vi "GUI_laptop v15 loop time characterization.vi"() -> ()   [LabVIEW 2019]
uses:
  <vilib>/Math Plots/3D Math Plots/3D Scatter/3D Scatter XCtrl/3D Scatter.xctl
  <vilib>/Platform/TimedLoop/XDataNode/timing_clust.ctl
  <vilib>/Platform/TimedLoop/XDataNode/nitl_modes.ctl
  <vilib>/Platform/TimedLoop/XDataNode/wakeup.ctl
  <vilib>/Analysis/_algsub.llb/Real Vector Norm.vi
  <vilib>/Instr/_visa.llb/VISA Configure Serial Port (Instr).vi
  <vilib>/Utility/file.llb/Write Delimited Spreadsheet (DBL).vi
  <vilib>/addons/System Identification/Data Preprocess.llb/SI Lowpass Filter (MISO Array).vi
  <vilib>/Math Plots/3D Math Plots/3D Scatter/3D Scatter Datatype/Public/Plot Helper (Vector).vi
  <vilib>/platform/TimedLoop/XDataNode/XDataNode.xnode
  <vilib>/Platform/TimedLoop/XDataNode/XDNodeRunTimeDep.lvlib
  <vilib>/Analysis/NI_AALPro.lvlib
  <vilib>/Math Plots/3D Math Plots/3D Scatter/3D Scatter Datatype/3D Scatter Datatype.lvclass
  <vilib>/addons/System Identification/NI_SysID.lvlib
panel:
  out "Frame Duration 2":i64
  out "Frame Duration":i64
  out "Period":i64
  out "Finished Late? [i-1] 3":bool
  out "Actual End [i-1] 2":i64
  out "Expected End [i-1] 2":i64
  out "Actual End [i-1]":i64
  out "Expected End [i-1]":i64
  out "Finished Late? [i-1] 2":bool
  in  "Motion scale L3 outside rcm":dbl=2.0
  in  "L5 Deadzone":dbl
  in  "Sample rate":u32=500
  in  "Cutoff Frequency":dbl=10.0
  in  "Motion scale L1 L2":dbl=10.0
  in  "Motion scale L3":dbl=2.0
  in  "Save Path 4":path=path "C:/Users/jimmy/Documents/GitHub/Arduino-LabVIEW/zhantao/read_data_abs_filtered.csv"
  in  "Save Path 3":path=path "C:/Users/jimmy/Documents/GitHub/Arduino-LabVIEW/zhantao/read_data_abs_sending.csv"
  out "stimulus signals out":dbl[][](array[numeric]) format="%.2f"
  in  "L5 Offset":dbl
  in  "L5 Scale":dbl=1.0
  in  "Motion Scale L4":dbl=30.0
  out "spreadsheet string":string
  in  "Save Path 2":path=path "C:/Users/jimmy/Documents/GitHub/Arduino-LabVIEW/zhantao/read_data_delt.csv"
  out "send values":dbl[](array[numeric])
  out "Robot Feedback (l1 l2 l3 l4)":dbl[](array[numeric])
  in  "UDP Send":bool
  in  "UDP Recv":bool
  in  "L5 bound":dbl=1000.0
  in  "L4 bound (deg)":dbl=1000.0
  in  "L3 bound (mm)":dbl=1000.0
  in  "L2 bound (deg)":dbl=1000.0
  in  "L1 bound (deg)":dbl=1000.0
  in  "Joystick Type":dbl(ring)=1.0 items=["Rigid Joystick", "Free Joystick"]
  out "Finished Late? [i-1]":bool
  in  "Epsilon":dbl=0.2
  out "3D Scatter":refnum<class "3D Plot Datatype.lvclass">[](xcontrol)
  out "Random Point":dbl[](array[numeric])
  out "Virtual Cursor":dbl[](array[numeric])
  out "Iteration Duration":i64
  in  "Num of Points":i32=10
  in  "z bound":dbl=2.0
  in  "y bound":dbl=5.0
  in  "x bound":dbl=5.0
  in  "Stop":bool
  in  "Round Decimals":dbl=2.0 format="%#_15g"
  in  "Save Data":bool
  in  "Save Path":path=path "C:/Users/jimmy/Documents/GitHub/Arduino-LabVIEW/zhantao/read_data_abs.csv"
  in  "x speed":dbl=0.5
  in  "z speed":dbl=0.5
  in  "y speed":dbl=0.5
  out "error out":errorcluster
  in  "baud rate":u32=250000
  in  "VISA resource name":refnum<visa-resource-name>
  # "Other stuff"
  # "Reading Commands"
  # "Joystick Selection"
  # "Plotting"
  # "Data Saving"
  # "Arduino Communication"
  # "Master Slave Communication"
  # "Parameters"
  # "TODO: add a lowpass filter for l5"
  # "TODO: fix the bounds; currently bounds are arbitrary"
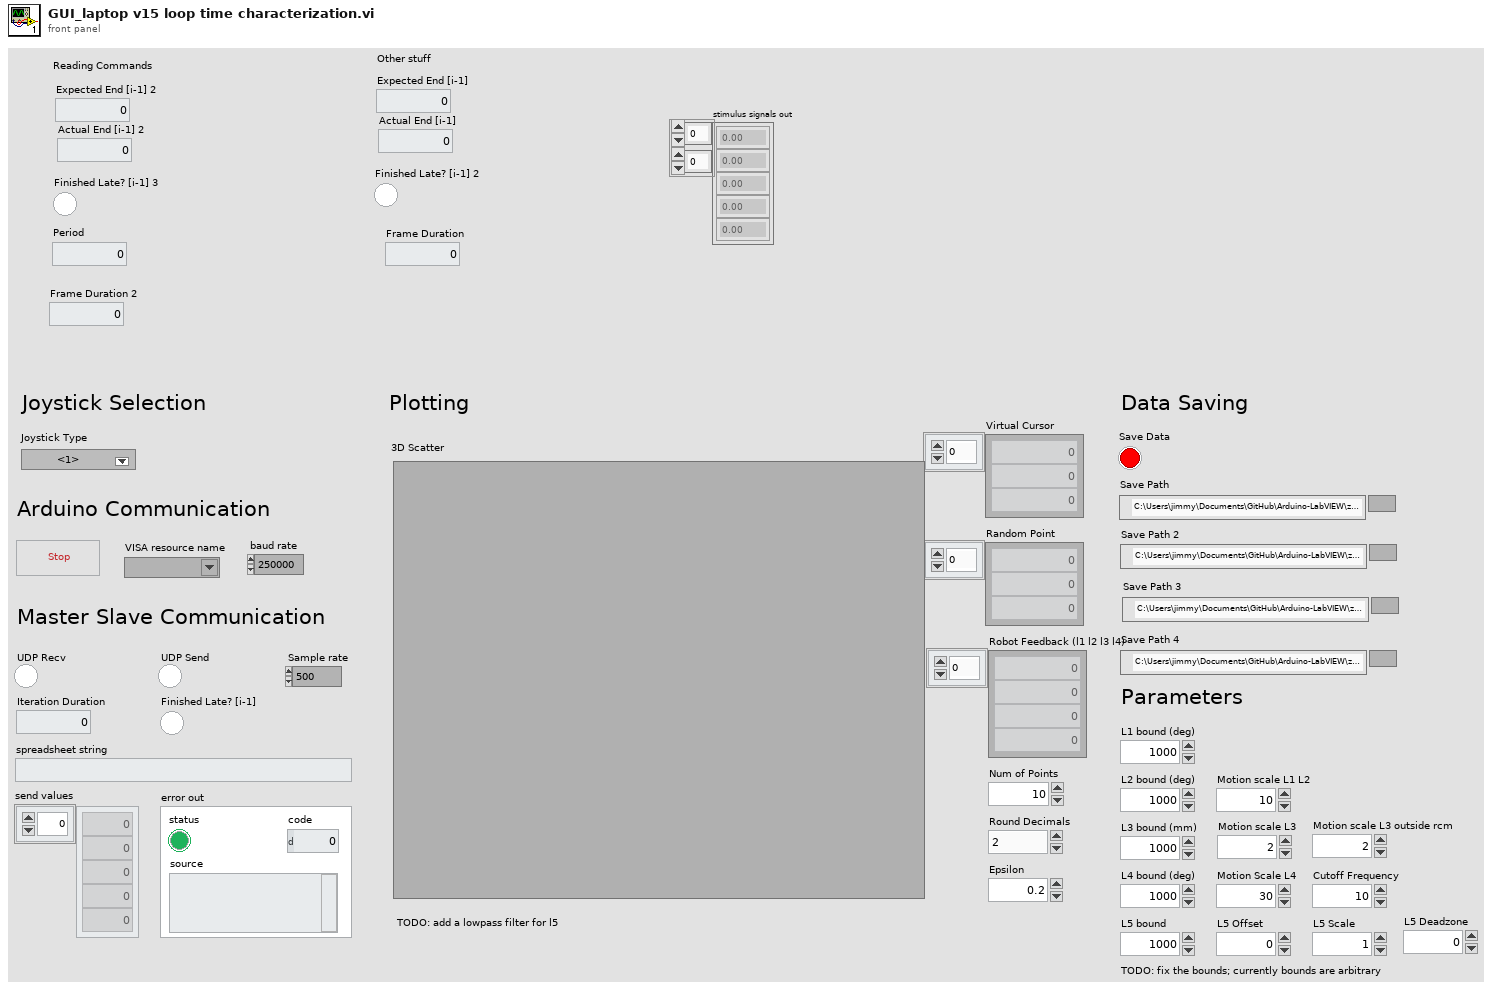
[diagram p1: front panel]
types:
  T1 = typedef "XDNodeRunTimeDep.lvlib/timing_clust.ctl" = cluster{"Expected End [f-1]":u64, "Actual End [f-1]":u64, "Finished Late? [f-1]":bool, "Expected End [i-1]":u64, "Actual End [i-1]":u64, "Finished Late? [i-1]":bool, "Expected Start [i]":u64, "Actual Start [i]":u64, "Expected Start [f]":u64, "Actual Start [f]":u64, "Source Name":string, "Structure Name":string, "Period":i64, "Deadline":i64, "Offset":i64, "Start":i64, "Priority":i32, "Timeout":i32, "Mode":T2, "Wakeup Reason":T3, "Error":errorcluster, "Source Type":string, "Secondary Source Type":string, "Global End Time":u64, "Global Start Time":u64, "Frame Duration":u64, "Iteration Duration":u64, "Assigned CPU":i32, "I/O Scan Engine Mode":u32}
  T2 = typedef "XDNodeRunTimeDep.lvlib/nitl_modes.ctl" = enum32{"No Change", "Process missed periods, maintain original phase", "Discard missed periods, maintain original phase", "Process missed periods, ignore original phase", "Discard missed periods, ignore original phase"}
  T3 = typedef "XDNodeRunTimeDep.lvlib/wakeup.ctl" = enum32{"Normal", "Aborted", "Asynchronous wakeup", "Timing source error", "Timed loop error", "Timeout"}
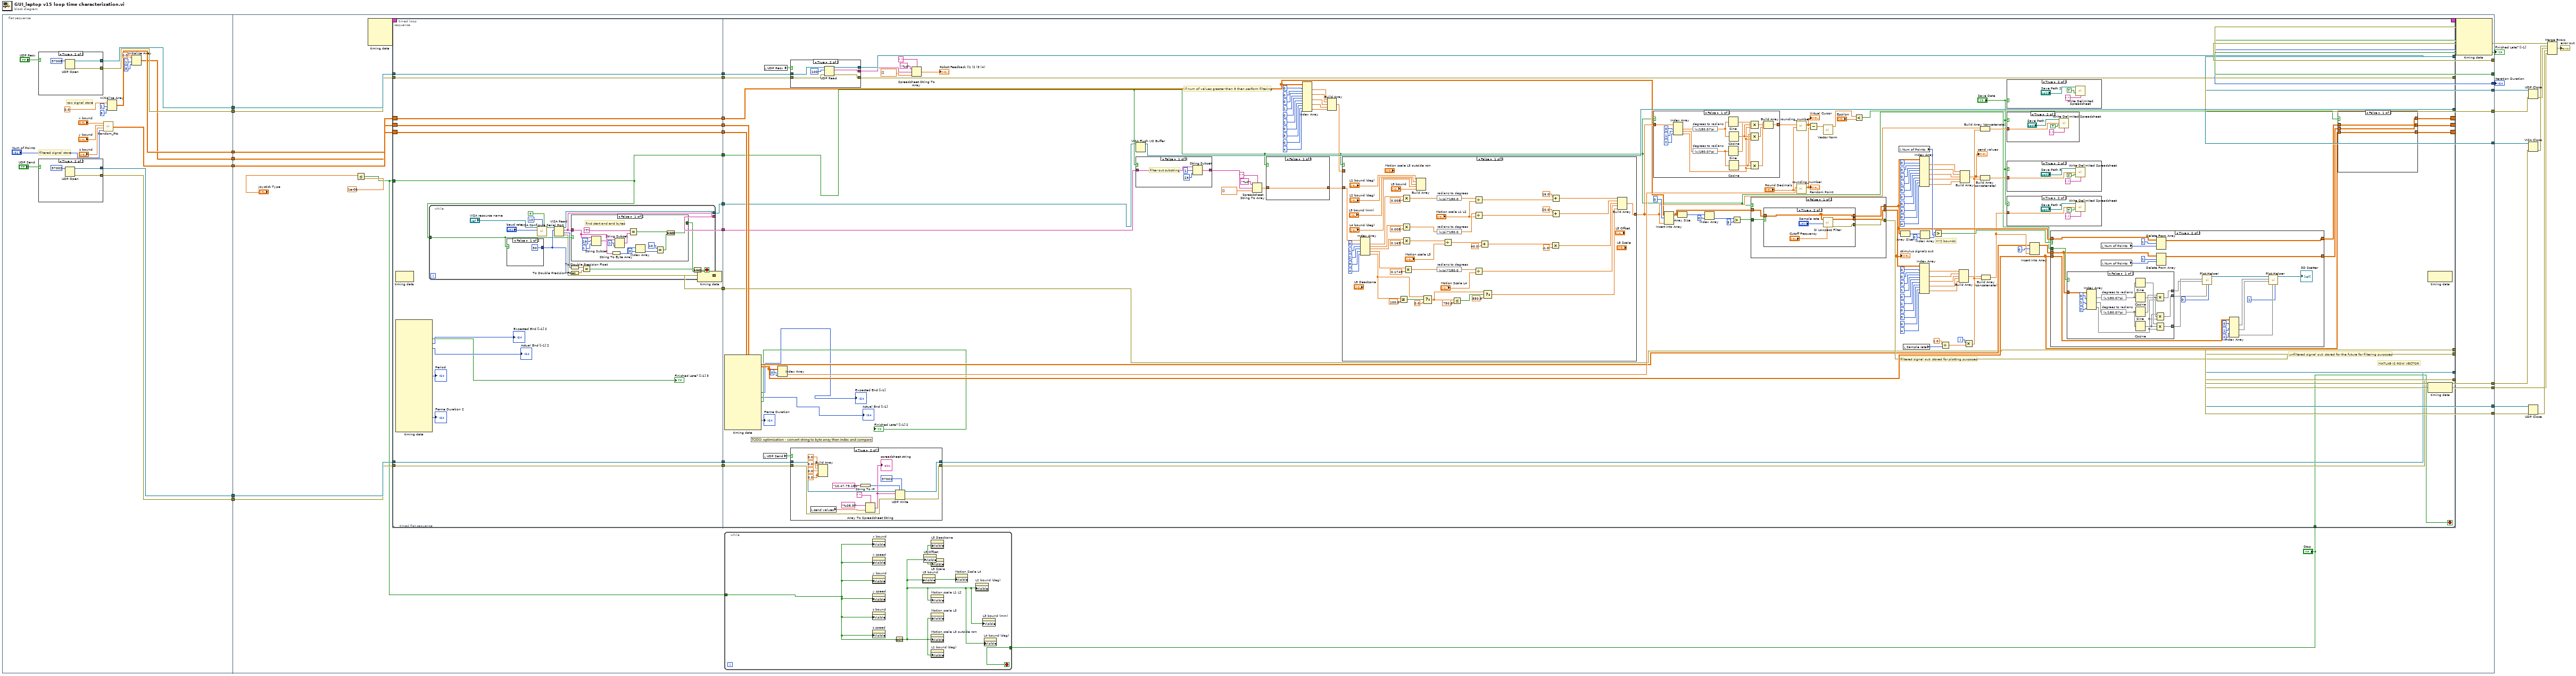
[diagram p0: block diagram]
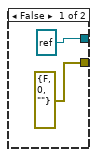
[diagram p2: hidden frame]
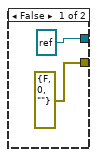
[diagram p3: hidden frame]
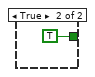
[diagram p4: hidden frame]
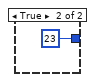
[diagram p5: hidden frame]
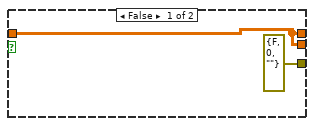
[diagram p8: hidden frame]
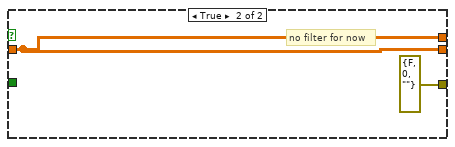
[diagram p9: hidden frame]
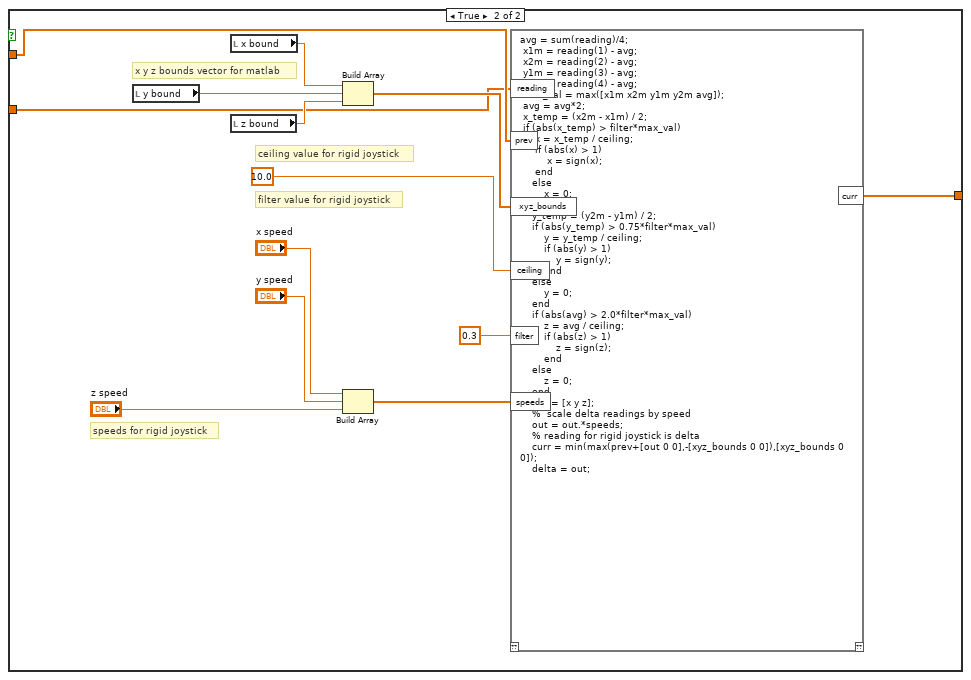
[diagram p10: hidden frame]
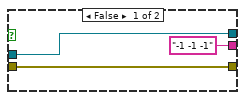
[diagram p13: hidden frame]
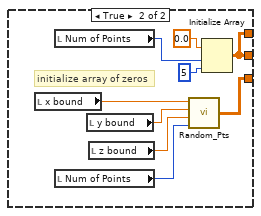
[diagram p15: hidden frame]
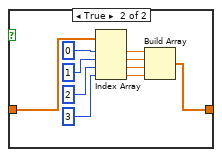
[diagram p17: hidden frame]
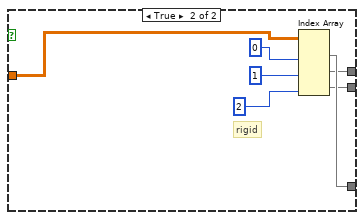
[diagram p20: hidden frame]
diagram:
  n1 = flat-sequence {
    tunnel: [w32] -> w18
    tunnel: [w36] -> w17
    tunnel: [w31] -> w16
    tunnel: [w30] -> w15
    tunnel: [w27] -> w14
    tunnel: [w26] -> w13
    tunnel: [w22] -> w2
    tunnel: [w71] -> w21
    tunnel: [w70] -> w20
    tunnel: [w68] -> w12
    tunnel: [w66] -> w19
    tunnel: w18 -> [w69]
    tunnel: w17 -> [w67]
    tunnel: w16 -> [w65]
    tunnel: w15 -> [w64]
    tunnel: w14 -> [w63]
    tunnel: w13 -> [w62]
    tunnel: [w61] -> w6
    tunnel: [w60] -> w11
    tunnel: [w59] -> w5
    tunnel: [w58] -> w4
    tunnel: [w57] -> w3
    tunnel: w2 -> [w56]
    tunnel: [w55] -> w1
    frame #0 {
      # "filtered signal store"
      # "raw signal store"
      n2 = case shown="True" "UDP Recv" {
        tunnel: [refnum<k16> refnum ("port") w49] -> w30
        tunnel: [errorcluster {"status"=FALSE, "code"=0, "source"=""} ("error out") w48] -> w27
        frame False {
        }
        frame True {
          n3 = UDP Open(11:u16 37008 ("port")) -> (port=w49:refnum<k16>, 0:w48:errorcluster)  [unwired: 4 in, 1 out]
        }
      }
      n4 = case shown="True" "UDP Send" {
        tunnel: [refnum<k16> refnum ("port") w44] -> w31
        tunnel: [errorcluster {"status"=FALSE, "code"=0, "source"=""} ("error out") w43] -> w26
        frame False {
        }
        frame True {
          n5 = UDP Open(11:u16 37002 ("port")) -> (port=w44:refnum<k16>, 0:w43:errorcluster)  [unwired: 4 in, 1 out]
        }
      }
      n6 = call "Random_Pts.vi"("Num of Points"="Num of Points", "z bound"="z bound", "y bound"="y bound", "x bound"="x bound") -> ("appended array"=w36:dbl[][])
      n7 = Initialize Array(0.0 ("element"), 1 ("dimension size"), 5 ("dimension size")) -> (w32:dbl[][])
      n8 = Initialize Array(0.0 ("element"), 1 ("dimension size"), 5 ("dimension size")) -> (w22:dbl[][])
    }
    frame #1 {
      n9 = Less Or Equal?(x="Joystick Type", y=1e-06) -> (x <= y?=w51:bool)
      n10 = node-c288() -> (w73:T1)  [unwired: 4 in]
      n11 = timed-loop {
        tunnel: [w95] -> w71
        tunnel: [w94] -> w70
        shift-right: [w83] -> _
        shift-left: w69 -> [w84]
        timing: w73 -> [_]
        timing-out: [_] -> w72
        shift-right: [w81] -> _
        shift-left: w67 -> [w82]
        tunnel: w65 -> [w93]
        tunnel: w64 -> [w92]
        tunnel: w63 -> [w91]
        tunnel: w62 -> [w90]
        tunnel: [w89] -> w61
        tunnel: [w88] -> w60
        tunnel: [w87] -> w59
        tunnel: [w86] -> w58
        tunnel: [w85] -> w57
        shift-right: [w79] -> _
        shift-left: w56 -> [w80]
        tunnel: "Stop" -> [w78]
        tunnel: w51 -> [w77]
        i -> [w199]
        stop <- w183 stop-if-true
        n12 = timed-sequence {
          timing: _ -> [_]
          timing-out: _ -> [_]
          tunnel: [w125] -> w95
          tunnel: [w124] -> w94
          tunnel: w93 -> [w123]
          tunnel: w92 -> [w122]
          tunnel: w91 -> [w121]
          tunnel: w90 -> [w120]
          tunnel: [w119] -> w89
          tunnel: [w118] -> w88
          tunnel: [w117] -> w87
          tunnel: [w116] -> w86
          tunnel: [w115] -> w85
          tunnel: w84 -> [w114]
          tunnel: [w113] -> w83
          tunnel: w82 -> [w112]
          tunnel: [w111] -> w81
          tunnel: w80 -> [w110]
          tunnel: [w109] -> w79
          tunnel: w78 -> [w97]
          tunnel: w77 -> [w96]
          n13 = timed-flat-sequence {
            tunnel: w110 -> [w135]
            tunnel: w112 -> [w136]
            tunnel: w114 -> [w137]
            tunnel: w120 -> [w138]
            tunnel: w121 -> [w139]
            tunnel: w122 -> [w140]
            tunnel: w123 -> [w141]
            tunnel: [w141] -> w108
            tunnel: [w140] -> w107
            tunnel: [w139] -> w106
            tunnel: [w138] -> w105
            tunnel: [w137] -> w104
            tunnel: [w136] -> w103
            tunnel: [w135] -> w102
            tunnel: [w134] -> w101
            tunnel: [w133] -> w100
            tunnel: [w132] -> w99
            tunnel: [w128] -> w98
            tunnel: w96 -> [w128]
            tunnel: [w254] -> w125
            tunnel: [w185] -> w124
            tunnel: [w262] -> w119
            tunnel: [w261] -> w118
            tunnel: [w260] -> w117
            tunnel: [w259] -> w116
            tunnel: [w244] -> w115
            tunnel: [w305] -> w113
            tunnel: [w301] -> w111
            tunnel: [w201] -> w109
            tunnel: w108 -> [w267]
            tunnel: w107 -> [w266]
            tunnel: w106 -> [w264]
            tunnel: w105 -> [w263]
            tunnel: w104 -> [w209]
            tunnel: w103 -> [w302]
            tunnel: w102 -> [w204]
            tunnel: w101 -> [w190]
            tunnel: w100 -> [w189]
            tunnel: w99 -> [w185]
            tunnel: w98 -> [w184]
            tunnel: w97 -> [w183]
            frame #0 {
              n14 = node-c288() -> (→"Finished Late? [i-1] 3":bool, →"Expected End [i-1] 2":i64, →"Actual End [i-1] 2":i64, →"Period":i64, →"Frame Duration 2":i64)  [unwired: 1 in, 18 out]
              n15 = while {
                tunnel: [w142] -> w133
                tunnel: [w155] -> w132
                tunnel: [w149] -> w134
                tunnel: w128 -> [w143]
                stop <- w145 stop-if-true
                n16 = case shown="False" w143 {
                  tunnel: [30 u32 23 ("byte count")] -> w148
                  frame False {
                  }
                  frame True {
                  }
                }
                n17 = call-poly "VISA Configure Serial Port"("VISA resource name"="VISA resource name", "termination char\n(0xA = '\\n' = LF)"=u8 10 ("termination char\n(0xA = '\\n' = LF)"), "Enable Termination\nChar (T)"=TRUE ("Enable Termination\nChar (T)"), "baud rate (9600)"="baud rate") -> ("VISA resource name out"=w150:refnum<visa-resource-name>)  [unwired: 10 in, 1 out]
                n18 = VISA Read(VISA resource name=w150, byte count=w148) -> (VISA resource name out=w149:refnum<visa-resource-name>, read buffer=w142:string, return count=w157:u32, error out=w155:errorcluster)  [unwired: 1 in]
                n19 = To Double Precision Float(number=w157) -> (double precision float=w156:dbl)
                n20 = To Double Precision Float(number=w148) -> (double precision float=w147:dbl)
                n21 = case shown="False" w143 {
                  tunnel: [w164 TRUE] -> w144
                  tunnel: w142 -> [w167 _]
                  frame False {
                    # "find start and end bytes"
                    n22 = String Subset(string=w167, offset (0)=29, length (rest)=1) -> (substring=w162:string)
                    n23 = String To Byte Array(string=w162) -> (unsigned byte array=w161:u8[])
                    n24 = String Subset(string=w167, length (rest)=1) -> (substring=w170:string)  [unwired: 1 in]
                    n25 = Equal?(x="T", y=w170) -> (x = y?=w166:bool)
                    n26 = Index Array(array=w161, index=0) -> (element=w159:u8)
                    n27 = Equal?(x=10, y=w159) -> (x = y?=w165:bool)
                    n28 = And(x=w166, y=w165) -> (x .and. y?=w164:bool)
                  }
                  frame True {
                  }
                }
                n29 = Equal?(x=w156, y=w147) -> (x = y?=w146:bool)
                n30 = And(x=w146, y=w144) -> (x .and. y?=w145:bool)
              }
              n31 = node-c288() -> ()  [unwired: 1 in, 1 out]
            }
            frame #1 {
              # "unfiltered signal out; stored for the future for filtering purposes"
              # "filtered signal out; stored for plotting purposes"
              # "XYZ bounds"
              # "if num of values greater than 5 then perform filtering"
              # "MATLAB IS ROW VECTOR"
              n32 = node-c288() -> (→"Expected End [i-1]":i64, →"Actual End [i-1]":i64, →"Finished Late? [i-1] 2":bool, →"Frame Duration":i64)  [unwired: 1 in, 11 out]
              n33 = local read "UDP Send"() -> (w194:bool)
              n34 = local read "UDP Recv"() -> (w265:bool)
              n35 = Index Array(array=w302, index (col)=0 ("index (row)")) -> (element=w276:dbl[])  [unwired: 1 in]
              n36 = case shown="True" w265 {
                tunnel: w266 -> [w413 w420]
                tunnel: w264 -> [w414 w419]
                tunnel: [w414 w418] -> w262
                tunnel: [w413 w417] -> w260
                tunnel: ["-1 -1 -1" w415] -> w255
                frame False {
                }
                frame True {
                  n37 = UDP Read(connection ID=w420, max size (548)=100, 8:w419) -> (data out=w415:string, error out=w418:errorcluster, 3:w417:refnum<k16>)  [unwired: 1 in, 2 out]
                }
              }
              n38 = case shown="True" w194 {
                tunnel: w267 -> [w395 w411]
                tunnel: w263 -> [w396 w407]
                tunnel: [w396 w403] -> w261
                tunnel: [w395 w402] -> w259
                frame False {
                }
                frame True {
                  w401 = 0.0 ("element")
                  n39 = local read "send values"() -> (w397:dbl[])
                  n40 = Build Array(0.0 ("element"), 0.0 ("element"), 0.0 ("element"), w401, w401) -> ()  [unwired: 1 out]
                  n41 = String To IP(1:"10.47.79.181" ("name")) -> (0:w405:u32)
                  n42 = Array To Spreadsheet String(delimiter (Tab)=" ", array=w397, 3:"%08.3f" ("format string")) -> (spreadsheet string=w408:string)
                  "spreadsheet string" <- w408
                  n43 = UDP Write(address=w405, port or service name=u16 37001, connection ID=w411, data in=w408, 8:w407) -> (error out=w403:errorcluster, 3:w402:refnum<k16>)  [unwired: 1 in]
                }
              }
              n44 = Spreadsheet String To Array(delimiter (Tab)=" ", format string="%d", spreadsheet string=w255, array type (2D Dbl)=dbl[] []) -> (array=→"Robot Feedback (l1 l2 l3 l4)":dbl[])
              n45 = VISA Flush I/O Buffer(VISA resource name=w190) -> (VISA resource name out=w254:refnum<visa-resource-name>)  [unwired: 2 in, 1 out]
              n46 = case shown="False" w184 {
                tunnel: w189 -> [w440 w441]
                tunnel: [w437 w441] -> w277
                frame False {
                  # "filter out substring"
                  n47 = String Subset(string=w440, offset (0)=1, length (rest)=29) -> (substring=w437:string)
                }
                frame True {
                }
              }
              n48 = Spreadsheet String To Array(delimiter (Tab)=",", format string="%d", spreadsheet string=w277, array type (2D Dbl)=dbl[] []) -> (array=w278:dbl[])
              n49 = case shown="False" w184 {
                tunnel: w278 -> [w442 w446]
                tunnel: [w442 w445] -> w252
                frame False {
                }
                frame True {
                  n50 = Index Array(array=w446, index #1=0 ("Plot ID"), index #2=1 ("Plot ID"), index #3=2 ("Plot ID"), index #4=3 ("index")) -> (element #1=w449:dbl, element #2=w448:dbl, element #3=w447:dbl, element #4=w443:dbl)
                  n51 = Build Array(w449, w448, w447, w443) -> (w445:dbl[])
                }
              }
              n52 = Index Array(array=w209, index (row) #1=0 ("disabled index (row)"), index (col) #1=0 ("disabled index (col)"), index (row) #2=0 ("disabled index (row)"), index (col) #2=1 ("disabled index (col)"), index (row) #3=0 ("disabled index (row)"), index (col) #3=2 ("disabled index (col)"), index (row) #4=0 ("disabled index (row)"), index (col) #4=3 ("disabled index (col)"), index (row) #5=0 ("disabled index (row)"), index (col) #5=4 ("disabled index (col)")) -> (element #1=w287:dbl, element #2=w286:dbl, element #3=w285:dbl, element #4=w280:dbl, element #5=w279:dbl)
              n53 = Build Array(w287, w286, w285, w280, w279) -> (w253:dbl[])
              n54 = case shown="False" w184 {
                tunnel: w253 -> [_ w381]
                tunnel: w252 -> [w368 w380]
                tunnel: [w328 w379] -> w228
                frame False {
                  n55 = Index Array(array=w368, index #1=0 ("Plot ID"), index #2=1 ("Plot ID"), index #3=2 ("Plot ID"), index #4=3 ("Plot ID"), index #5=4 ("Plot ID")) -> (element #1=w367:dbl, element #2=w355:dbl, element #3=w347:dbl, element #4=w345:dbl, element #5=w337:dbl)
                  n56 = Greater Or Equal?(x=w337, y=100.0) -> (x >= y?=w335:bool)
                  n57 = Multiply(x=w367, y=0.005) -> (x*y=w363:dbl)
                  n58 = Multiply(x=w355, y=0.005) -> (x*y=w358:dbl)
                  n59 = Multiply(x=w347, y=0.163) -> (x*y=w351:dbl)
                  n60 = Multiply(x=w345, y=0.1745) -> (x*y=w344:dbl)
                  n61 = Build Array("L1 bound (deg)", "L2 bound (deg)", "L3 bound (mm)", "L4 bound (deg)", "L5 bound") -> ()  [unwired: 1 out]
                  n62 = Select(t=w337, s=w335, f=0.0) -> (s? t:f=w330:dbl)
                  n63 = expression code="(x/pi)*180.0" "radians to degrees"(w363) -> (w362:dbl)
                  n64 = expression code="(x/pi)*180.0" "radians to degrees"(w358) -> (w357:dbl)
                  n65 = expression code="(x/pi)*180.0" "radians to degrees"(w344) -> (w343:dbl)
                  n66 = Divide(x=w351, y="Motion scale L3") -> (x/y=w349:dbl)
                  n67 = Less Or Equal?(x=w330, y=750.0) -> (x <= y?=w331:bool)
                  n68 = Divide(x=w362, y="Motion scale L1 L2") -> (x/y=w365:dbl)
                  n69 = Divide(x=w357, y="Motion scale L1 L2") -> (x/y=w360:dbl)
                  n70 = Divide(x=w343, y="Motion Scale L4") -> (x/y=w338:dbl)
                  n71 = Add(x=w349, y=40.0) -> (x+y=w353:dbl)
                  n72 = Select(t=w330, s=w331, f=850.0) -> (s? t:f=w329:dbl)
                  n73 = Multiply(x=w353, y=-1.0) -> (x*y=w339:dbl)
                  n74 = Add(x=16.0, y=w365) -> (x+y=w341:dbl)
                  n75 = Add(x=20.0, y=w360) -> (x+y=w340:dbl)
                  n76 = Build Array(w341, w340, w339, w338, w329) -> (w328:dbl[])
                }
                frame True {
                  # "ceiling value for rigid joystick"
                  # "filter value for rigid joystick"
                  # "speeds for rigid joystick"
                  # "x y z bounds vector for matlab"
                  n77 = local read "y bound"() -> (w390:dbl)
                  n78 = local read "x bound"() -> (w389:dbl)
                  n79 = local read "z bound"() -> (w391:dbl)
                  n80 = Build Array(w389, w390, w391) -> (w382:dbl[])
                  n81 = Build Array("x speed", "y speed", "z speed") -> (w385:dbl[])
                  n82 = script code="avg = sum(reading)/4;\n x1m = reading(1) - avg;\n x2m = reading(2) - avg;\n y1m = reading(3) - avg;\n y2m = reading(4) - avg;\n max_val = max([x1m x2m y1m y2m avg]);\n avg = avg*2;\n x_temp = (x2m - x1m) / 2;\n if (abs(x_temp) > filter*max_val)\n     x = x_temp / ceiling;\n     if (abs(x) > 1)\n         x = sign(x);\n     end\n    else\n        x = 0;\n    end\n    y_temp = (y2m - y1m) / 2;\n    if (abs(y_temp) > 0.75*filter*max_val)\n        y = y_temp / ceiling;\n        if (abs(y) > 1)\n            y = sign(y);\n        end\n    else\n        y = 0;\n    end\n    if (abs(avg) > 2.0*filter*max_val)\n        z = avg / ceiling;\n        if (abs(z) > 1)\n            z = sign(z);\n        end\n    else\n        z = 0;\n    end\n    out = [x y z];\n    %  scale delta readings by speed\n    out = out.*speeds;\n    % reading for rigid joystick is delta\n    curr = min(max(prev+[out 0 0],-[xyz_bounds 0 0]),[xyz_bounds 0 0]);\n    delta = out;"("xyz_bounds"=w382, "ceiling"=10.0 ("Real"), "filter"=0.3 ("Real"), "speeds"=w385, "reading"=w380, "prev"=w381) -> ("curr"=w379:dbl[])  [unwired: 1 in, 1 out]
                }
              }
              n83 = case shown="False" w184 {
                tunnel: [w466 w470] -> w303
                tunnel: w228 -> [w465 w470]
                frame False {
                  n84 = Index Array(array=w465, index #1=0 ("Plot ID"), index #2=1 ("Plot ID"), index #3=2 ("Plot ID")) -> (element #1=w464:dbl, element #2=w463:dbl, element #3=w453:dbl)
                  n85 = expression code="(x/180.0)*pi" "degrees to radians"(w464) -> (w462:dbl)
                  n86 = expression code="(x/180.0)*pi" "degrees to radians"(w463) -> (w461:dbl)
                  n87 = Sine(x=w462) -> (sin(x)=w459:dbl)
                  n88 = Sine(x=w461) -> (sin(x)=w458:dbl)
                  n89 = Cosine(x=w462) -> (cos(x)=w455:dbl)
                  n90 = Cosine(x=w461) -> (cos(x)=w456:dbl)
                  n91 = Compound Arithmetic op=MULTIPLY(w458, w455, w453) -> (w457:dbl)
                  n92 = Compound Arithmetic op=MULTIPLY(w456, w455, w453) -> (w454:dbl)
                  n93 = Compound Arithmetic op=MULTIPLY(w459, w456, w453) -> (w460:dbl)
                  n94 = Build Array(w460, w457, w454) -> (w466:dbl[])
                }
                frame True {
                }
              }
              n95 = Insert Into Array(array=w209, index (row)=0, new element=w228) -> (w245:dbl[][])  [unwired: 1 in]
              n96 = Array Size(array=w245) -> (size(s)=w248:i32[])
              n97 = Index Array(array=w248, index=0) -> (element=w247:i32)
              n98 = Greater?(x=w247, y=5) -> (0:w195:bool)
              n99 = case shown="False" w184 {
                tunnel: w195 -> [w316 _]
                tunnel: w245 -> [w318 w326]
                tunnel: [w317 w326] -> w207
                tunnel: [w315 errorcluster {"status"=FALSE, "code"=0, "source"=""} ("error out")] -> w244
                tunnel: [w314 w326] -> w210
                frame False {
                  n100 = case shown="True" w316 {
                    tunnel: w318 -> [w319 w324]
                    tunnel: [w319 w324] -> w317
                    tunnel: [errorcluster {"status"=FALSE, "code"=0, "source"=""} ("error out") w325] -> w315
                    tunnel: [w319 w323] -> w314
                    frame False {
                    }
                    frame True {
                      n101 = call-poly <vilib>:"SI Lowpass Filter.vi"("cutoff frequency"="Cutoff Frequency", "sampling rate (Hz)"="Sample rate", "stimulus signals in"=w324) -> ("error out"=w325:errorcluster, "stimulus signals out"=w323:dbl[][])  [unwired: 6 in, 1 out]
                    }
                  }
                }
                frame True {
                  # "no filter for now"
                }
              }
              "stimulus signals out" <- w210
              n102 = call "rounding_number.vi"("power of ten"="Round Decimals", "Array"=w303) -> ("rounded"=w274:dbl[])  [unwired: 9 in]
              "Virtual Cursor" <- w274
              n103 = call "rounding_number.vi"("power of ten"="Round Decimals", "Array"=w276) -> ("rounded"=w273:dbl[])  [unwired: 9 in]
              "Random Point" <- w273
              n104 = Subtract(x=w274, y=w273) -> (x-y=w272:dbl[])
              n105 = call-poly <vilib>:"Vector Norm.vi"("Input Vector"=w272) -> ("norm"=w271:dbl)  [unwired: 9 in, 1 out]
              n106 = Less?(x=w271, y="Epsilon") -> (x < y?=w269:bool)
              n107 = local read "Num of Points"() -> (w289:i32)
              n108 = Array Size(array=w207) -> (size(s)=w251:i32[])
              n109 = local read "Sample rate"() -> (w196:u32)
              n110 = Index Array(array=w207, index (row) #1=0 ("disabled index (col)"), index (col) #1=0 ("disabled index (row)"), index (row) #2=0 ("disabled index (col)"), index (col) #2=1 ("disabled index (row)"), index (row) #3=0 ("disabled index (col)"), index (col) #3=2 ("disabled index (row)"), index (row) #4=0 ("disabled index (col)"), index (col) #4=3 ("disabled index (row)"), index (row) #5=0 ("disabled index (col)"), index (col) #5=4 ("disabled index (col)")) -> (element #1=w233:dbl, element #2=w232:dbl, element #3=w231:dbl, element #4=w230:dbl, element #5=w229:dbl)
              n111 = Index Array(array=w210, index (row) #1=0 ("disabled index (col)"), index (col) #1=0 ("disabled index (row)"), index (row) #2=0 ("disabled index (col)"), index (col) #2=1 ("disabled index (row)"), index (row) #3=0 ("disabled index (col)"), index (col) #3=2 ("disabled index (row)"), index (row) #4=0 ("disabled index (col)"), index (col) #4=3 ("disabled index (row)"), index (row) #5=0 ("disabled index (col)"), index (col) #5=4 ("disabled index (col)")) -> (element #1=w216:dbl, element #2=w215:dbl, element #3=w214:dbl, element #4=w213:dbl, element #5=w212:dbl)
              n112 = Index Array(array=w251, index=0) -> (element=w290:i32)
              n113 = Greater?(x=w290, y=w289) -> (0:w288:bool)
              n114 = Divide(x=1.0, y=w196) -> (x/y=w197:dbl)
              n115 = Build Array(w216, w215, w214, w213, w212) -> (w193:dbl[])
              n116 = Build Array(w233, w232, w231, w230, w229) -> (w192:dbl[])
              "send values" <- w192
              n117 = Multiply(x=w199, y=w197) -> (x*y=w200:dbl)
              n118 = Build Array (concatenate)(w228, w200) -> (w227:dbl[])
              n119 = Build Array (concatenate)(w192, w200) -> (w208:dbl[])
              n120 = Build Array (concatenate)(w193, w200) -> (w205:dbl[])
              n121 = case shown="True" "Save Data" {
                frame False {
                }
                frame True {
                  n122 = call-poly <vilib>:"Write Delimited Spreadsheet.vi"("file path (dialog if empty)"="Save Path 2", "append to file? (new file:F)"=TRUE, "delimiter (\\t)"="," ("delimiter (\\t)")) -> ()  [unwired: 11 in, 2 out]
                }
              }
              n123 = case shown="True" "Save Data" {
                tunnel: w227 -> [_ w421]
                frame False {
                }
                frame True {
                  n124 = call-poly <vilib>:"Write Delimited Spreadsheet.vi"("file path (dialog if empty)"="Save Path", "1D data"=w421, "append to file? (new file:F)"=TRUE, "delimiter (\\t)"="," ("delimiter (\\t)")) -> ()  [unwired: 10 in, 2 out]
                }
              }
              n125 = case shown="True" "Save Data" {
                tunnel: w208 -> [_ w310]
                frame False {
                }
                frame True {
                  n126 = call-poly <vilib>:"Write Delimited Spreadsheet.vi"("file path (dialog if empty)"="Save Path 3", "1D data"=w310, "append to file? (new file:F)"=TRUE, "delimiter (\\t)"="," ("delimiter (\\t)")) -> ()  [unwired: 10 in, 2 out]
                }
              }
              n127 = case shown="True" "Save Data" {
                tunnel: w205 -> [_ w306]
                frame False {
                }
                frame True {
                  n128 = call-poly <vilib>:"Write Delimited Spreadsheet.vi"("file path (dialog if empty)"="Save Path 4", "1D data"=w306, "append to file? (new file:F)"=TRUE, "delimiter (\\t)"="," ("delimiter (\\t)")) -> ()  [unwired: 10 in, 2 out]
                }
              }
              n129 = Insert Into Array(array=w204, index (row)=0, new element=w205) -> (w203:dbl[][])  [unwired: 1 in]
              n130 = case shown="True" w288 {
                tunnel: w207 -> [w472 w494]
                tunnel: [w472 w493] -> w304
                tunnel: w302 -> [w471 w492]
                tunnel: w184 -> [_ w477]
                tunnel: w203 -> [_ w474]
                tunnel: [w471 w473] -> w202
                frame False {
                }
                frame True {
                  n131 = case shown="False" w477 {
                    tunnel: w474 -> [w511 w515]
                    tunnel: [w498 w514] -> w483
                    tunnel: [w497 w513] -> w482
                    tunnel: [w496 w512] -> w481
                    frame False {
                      n132 = Index Array(array=w511, index (col) #1=0 ("Plot ID"), index (col) #2=1 ("Plot ID"), index (col) #3=2 ("Plot ID")) -> (element #1=w501:dbl[], element #2=w500:dbl[], element #3=w499:dbl[])  [unwired: 3 in]
                      n133 = expression code="(x/180.0)*pi" "degrees to radians"(w501) -> (w507:dbl[])
                      n134 = expression code="(x/180.0)*pi" "degrees to radians"(w500) -> (w506:dbl[])
                      n135 = Sine(x=w507) -> (sin(x)=w505:dbl[])
                      n136 = Cosine(x=w507) -> (cos(x)=w502:dbl[])
                      n137 = Sine(x=w506) -> (sin(x)=w504:dbl[])
                      n138 = Cosine(x=w506) -> (cos(x)=w503:dbl[])
                      n139 = Compound Arithmetic op=MULTIPLY(w504, w502, w499) -> (w497:dbl[])
                      n140 = Compound Arithmetic op=MULTIPLY(w503, w502, w499) -> (w496:dbl[])
                      n141 = Compound Arithmetic op=MULTIPLY(w505, w503, w499) -> (w498:dbl[])
                    }
                    frame True {
                      # "rigid"
                      n142 = Index Array(array=w515, index (col) #1=0 ("disabled index (col)"), index (col) #2=1 ("index (col)"), index (col) #3=2 ("index (col)")) -> (element #1=w514:dbl[], element #2=w513:dbl[], element #3=w512:dbl[])  [unwired: 3 in]
                    }
                  }
                  n143 = local read "Num of Points"() -> (w491:i32)
                  n144 = local read "Num of Points"() -> (w476:i32)
                  n145 = Delete From Array(array=w494, length=1, index (row)=w491) -> (array with subset deleted=w493:dbl[][])  [unwired: 1 in, 1 out]
                  n146 = Delete From Array(array=w474, length=1, index (row)=w476) -> (array with subset deleted=w473:dbl[][])  [unwired: 1 in, 1 out]
                  n147 = call-poly <vilib>:"Plot Helper.vi"("Plot ID"=0, "z vector"=w481, "y vector"=w482, "x vector"=w483) -> ("3D Plot lvclass Array out"=w485:refnum<class "3D Plot Datatype.lvclass">[])  [unwired: 2 in, 5 out]
                  n148 = Index Array(array=w492, index (row) #1=0 ("index (row)"), index (row) #2=1 ("index (row)"), index (row) #3=2 ("index (row)")) -> (element #1=w489:dbl[], element #2=w488:dbl[], element #3=w487:dbl[])  [unwired: 3 in]
                  n149 = call-poly <vilib>:"Plot Helper.vi"("Plot ID"=1, "z vector"=w487, "y vector"=w488, "x vector"=w489, "3D Plot lvclass Array in"=w485) -> ("3D Plot lvclass Array out"=→"3D Scatter":refnum<class "3D Plot Datatype.lvclass">[])  [unwired: 1 in, 5 out]
                }
              }
              n150 = case shown="False" w269 {
                tunnel: w302 -> [w427 _]
                tunnel: [w427 w432] -> w301
                tunnel: w304 -> [w426 _]
                tunnel: [w426 w428] -> w305
                tunnel: w202 -> [w425 _]
                tunnel: [w425 w428] -> w201
                frame False {
                }
                frame True {
                  # "initialize array of zeros"
                  n151 = local read "x bound"() -> (w436:dbl)
                  n152 = local read "Num of Points"() -> (w430:i32)
                  n153 = local read "Num of Points"() -> (w433:i32)
                  n154 = local read "y bound"() -> (w435:dbl)
                  n155 = local read "z bound"() -> (w434:dbl)
                  n156 = call "Random_Pts.vi"("Num of Points"=w433, "z bound"=w434, "y bound"=w435, "x bound"=w436) -> ("appended array"=w432:dbl[][])
                  n157 = Initialize Array(0.0 ("element"), w430, 5 ("dimension size")) -> (w428:dbl[][])
                }
              }
              n158 = node-c288() -> ()  [unwired: 1 in, 1 out]
            }
          }
        }
        n159 = node-c288() -> ()  [unwired: 1 in, 1 out]
        n160 = node-c288() -> ()  [unwired: 1 in, 1 out]
      }
      n161 = while {
        tunnel: "Stop" -> [w75]
        tunnel: w51 -> [w74]
        stop <- w75 stop-if-true
        n162 = property on="x bound" class="DigNum (strict)"("Visible"=w74) -> ()  [unwired: 2 in, 2 out]
        n163 = property on="x speed" class="DigNum (strict)"("Visible"=w74) -> ()  [unwired: 2 in, 2 out]
        n164 = property on="y bound" class="DigNum (strict)"("Visible"=w74) -> ()  [unwired: 2 in, 2 out]
        n165 = property on="y speed" class="DigNum (strict)"("Visible"=w74) -> ()  [unwired: 2 in, 2 out]
        n166 = property on="z bound" class="DigNum (strict)"("Visible"=w74) -> ()  [unwired: 2 in, 2 out]
        n167 = property on="z speed" class="DigNum (strict)"("Visible"=w74) -> ()  [unwired: 2 in, 2 out]
        n168 = Not(x=w74) -> (.not. x?=w76:bool)
        n169 = property on="L5 bound" class="DigNum (strict)"("Visible"=w76) -> ()  [unwired: 2 in, 2 out]
        n170 = property on="L5 Offset" class="DigNum (strict)"("Visible"=w76) -> ()  [unwired: 2 in, 2 out]
        n171 = property on="L5 Deadzone" class="DigNum (strict)"("Visible"=w76) -> ()  [unwired: 2 in, 2 out]
        n172 = property on="L5 Scale" class="DigNum (strict)"("Visible"=w76) -> ()  [unwired: 2 in, 2 out]
        n173 = property on="Motion scale L1 L2" class="DigNum (strict)"("Visible"=w76) -> ()  [unwired: 2 in, 2 out]
        n174 = property on="Motion scale L3" class="DigNum (strict)"("Visible"=w76) -> ()  [unwired: 2 in, 2 out]
        n175 = property on="Motion scale L3 outside rcm" class="DigNum (strict)"("Visible"=w76) -> ()  [unwired: 2 in, 2 out]
        n176 = property on="L1 bound (deg)" class="DigNum (strict)"("Visible"=w76) -> ()  [unwired: 2 in, 2 out]
        n177 = property on="Motion Scale L4" class="DigNum (strict)"("Visible"=w76) -> ()  [unwired: 2 in, 2 out]
        n178 = property on="L2 bound (deg)" class="DigNum (strict)"("Visible"=w76) -> ()  [unwired: 2 in, 2 out]
        n179 = property on="L3 bound (mm)" class="DigNum (strict)"("Visible"=w76) -> ()  [unwired: 2 in, 2 out]
        n180 = property on="L4 bound (deg)" class="DigNum (strict)"("Visible"=w76) -> ()  [unwired: 2 in, 2 out]
      }
      n181 = node-c288(w72) -> (w68:errorcluster, w55:bool, w66:i64)  [unwired: 3 out]
    }
  }
  n182 = UDP Close(connection ID=w5, 8:w6) -> (error out=w9:errorcluster)  [unwired: 1 out]
  n183 = VISA Close(VISA resource name=w21, error in (no error)=w20) -> (error out=w10:errorcluster)
  n184 = UDP Close(connection ID=w4, 8:w11) -> (error out=w8:errorcluster)  [unwired: 1 out]
  n185 = Merge Errors(w12, w10, w9, w8, w3) -> (→"error out":errorcluster)
  "Iteration Duration" <- w19
  "Finished Late? [i-1]" <- w1
